vi "Re-Send Add file.vi"(6 "Milliseconds To Wait":i32=1000, 7 "Message Priority (Normal)":T1=enum."Normal", 8 "error in (no error)":errorcluster, 9 "Insert in front":bool, 10 "File Path Control":path, 11 "Message Enqueuer":refnum<class "Message Enqueuer.lvclass">) -> (0 "error out":errorcluster, 3 "Message Enqueuer out":refnum<class "Message Enqueuer.lvclass">)   [LabVIEW 2015, in "Add file Msg.lvclass"]
doc: "This VI sends the message to an actor."
uses:
  Add file Msg.lvclass
  <vilib>/ActorFramework/Message Enqueuer/Message Enqueuer.lvclass
  <vilib>/ActorFramework/Message Enqueuer/Message Priority.ctl
  Add file Msg.lvclass/Add file Msg.ctl
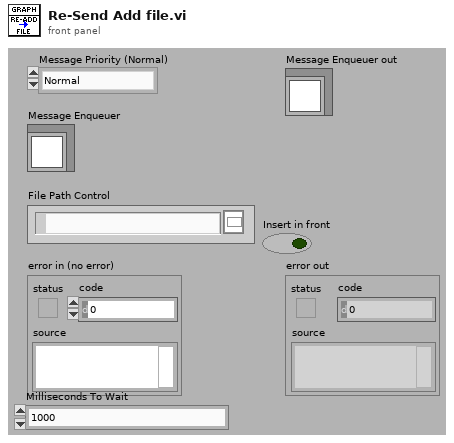
[diagram p1: front panel]
types:
  T1 = typedef "Actor Framework.lvlib/Message Enqueuer.lvclass/Message Priority.ctl" = enum16{"Low", "Normal", "High"}
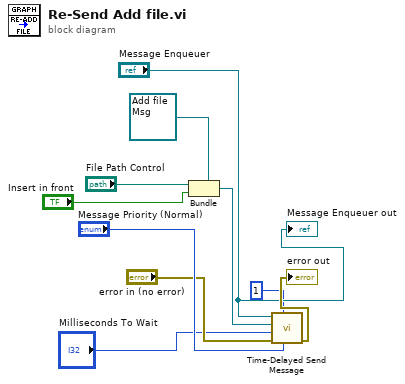
[diagram p0: block diagram]
diagram:
  n1 = Bundle(cluster=refnum<class "Add file Msg.lvclass"> refnum ("Object"), "File Path Control", "Insert in front") -> (w7:refnum<class "Add file Msg.lvclass">)
  n2 = call <vilib>:"Time-Delayed Send Message.vi"("Message Priority (Normal)"="Message Priority (Normal)", "# Copies (0 = infinite repeat)"=u32 1, "error in (no error)"="error in (no error)", "Milliseconds To Wait"="Milliseconds To Wait", "Message"=w7, "Message Enqueuer"="Message Enqueuer") -> ("error out"=→"error out":errorcluster)  [unwired: 4 in, 1 out]
  "Message Enqueuer out" <- "Message Enqueuer"
